vi "DTACQ - Set Data Size.vi"(8 "error in":errorcluster, 9 "Data Size":T1, 10 "Module Type":T2=enum."Analog In Module", 11 "Address":string) -> (0 "error out":errorcluster, 2 "Acknowledged":bool)   [LabVIEW 2017, in "Communications Library.lvlib"]
doc: "Set the data type used by all modules of the specified type (eg. set all analog in modules to receive 32 bit numbers)"
uses:
  Communications Library.lvlib
  Typedefs/DTACQ Device Type--Enum.ctl
  Typedefs/Data Size--Enum.ctl
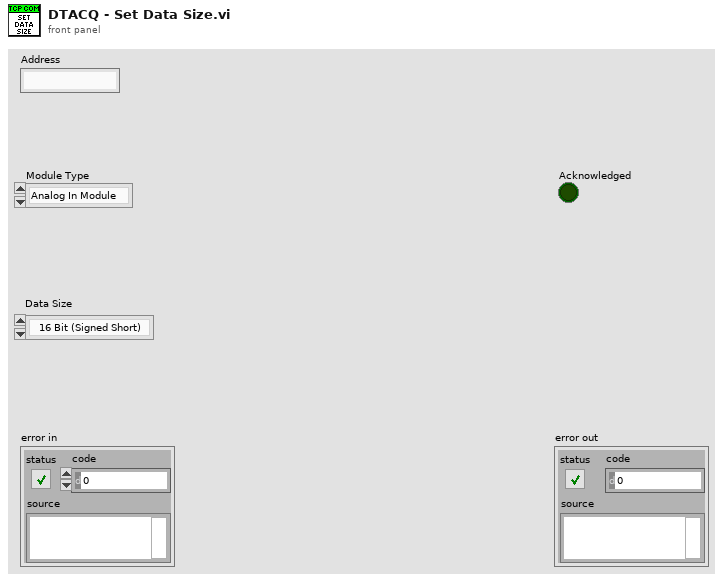
[diagram p1: front panel]
types:
  T1 = typedef "Communications Library.lvlib/Data Size--Enum.ctl" = enum16{"16 Bit (Signed Short)", "32 Bit (Signed Long)"}
  T2 = typedef "Communications Library.lvlib/DTACQ Device Type--Enum.ctl" = enum16{"Carrier", "Analog In Module", "Analog Out Module", "Generic Module"}
  T3 = typedef "Communications Library.lvlib/DTACQ Module Configuration--Cluster.ctl" = cluster{"Name":string, "Position":string, "Module Type":T2, "Control Port":i32, "Timeout (ms)":i32, "Channels":i32}
  T4 = typedef "Communications Library.lvlib/DTACQ Connection Data--Cluster.ctl" = cluster{"Description":string, "Address":string, "Port":u16, "timeout (ms)":i32, "Termination Character":string, "TCP Connection Reference":refnum<k5>, "Open Connection":bool}
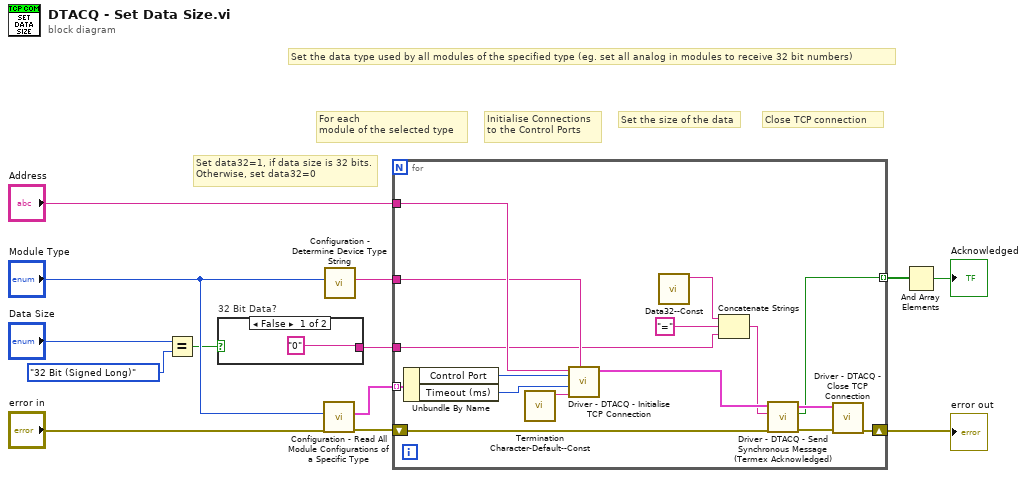
[diagram p0: block diagram]
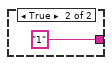
[diagram p2: hidden frame]
diagram:
  # "For each \nmodule of the selected type"
  # "Set data32=1, if data size is 32 bits.\nOtherwise, set data32=0"
  # "Set the data type used by all modules of the specified type (eg. set all analog in modules to receive 32 bit numbers)"
  # "Close TCP connection"
  # "Set the size of the data"
  # "Initialise Connections\nto the Control Ports"
  n1 = Equal?(x="Data Size", y=Data_Size--Enum."32 Bit (Signed Long)") -> (x = y?=w4:bool)
  n2 = case "32 Bit Data?" shown="False" w4 {
    tunnel: ["0" "1"] -> w3
    frame False {
    }
    frame True {
    }
  }
  n3 = call "Configuration - Read All Module Configurations of a Specific Type.vi"("error in"="error in", "Module Type"="Module Type") -> ("error out"=w7:errorcluster, "Module Configurations"=w9:T3[])  [unwired: 7 in, 1 out]
  n4 = call "Configuration - Determine Device Type String.vi"("Device Type In"="Module Type") -> ("Type String Out"=w10:string)  [unwired: 10 in]
  n5 = for {
    tunnel: "Address" -> [w31]
    tunnel: w10 -> [w28]
    shift-right: [w29] -> w12
    shift-left: w7 -> [w24]
    tunnel: w9 -> [w27] mode=indexing
    tunnel: w3 -> [w20]
    tunnel: [w16] -> w2 mode=indexing
    n6 = Unbundle By Name(w27) -> ("Control Port"=w26:i32, "Timeout (ms)"=w25:i32)
    n7 = call "Termination Character-Default--Const.vi"() -> ("Termination Character"=w30:string)  [unwired: 11 in]
    n8 = call "Driver - DTACQ - Initialise TCP Connection.vi"("Description"=w28, "Termination Character"=w30, "timeout (ms)"=w25, "Port"=w26, "Address"=w31) -> ("DTACQ Connection Data Out"=w23:T4)  [unwired: 6 in]
    n9 = call "Data32--Const.vi"() -> ("Data32 Command"=w22:string)  [unwired: 11 in]
    n10 = Concatenate Strings(w22, "=" ("string"), w20) -> (w19:string)
    n11 = call "Driver - DTACQ - Send Synchronous Message (Termex Acknowledged).vi"("error in"=w24, "Message to Send"=w19, "DTACQ Connection Data In"=w23) -> ("error out"=w18:errorcluster, "Message Acknowledged"=w16:bool, "DTACQ Connection Data Out"=w17:T4)  [unwired: 5 in, 1 out]
    n12 = call "Driver - DTACQ - Close TCP Connection.vi"("error in"=w18, "DTACQ Connection Data In"=w17) -> ("error out"=w29:errorcluster)  [unwired: 8 in, 1 out]
  }
  "error out" <- w12
  n13 = And Array Elements(Boolean array=w2) -> (logical AND=→"Acknowledged":bool)
